vi "Get Error Type.vi"(1 "Newly Reported Error":T4, 2 "Last (latest) Handled Error":T2) -> (0 "Error Type":T1)   [LabVIEW 2023, in "Error Manager.lvlib"]
doc: "Blank VI with error handling."
uses:
  Error Manager.lvlib
  Reported Error (cluster).ctl
  Public API VIs/Pop-up New Error Dialogue Instruction (enum).ctl
  Handled Error (cluster).ctl
  Read-Unread Status (enum).ctl
  Error Log/Error Type (enum).ctl
  Error Log/Error Log.lvclass
panel:
  # "Input\nInputs to the VI"
  # "Development\nControls or indicators that are useful for development or testing, but which are not outputs of the VI."
  # "Output\nOutputs of the VI"
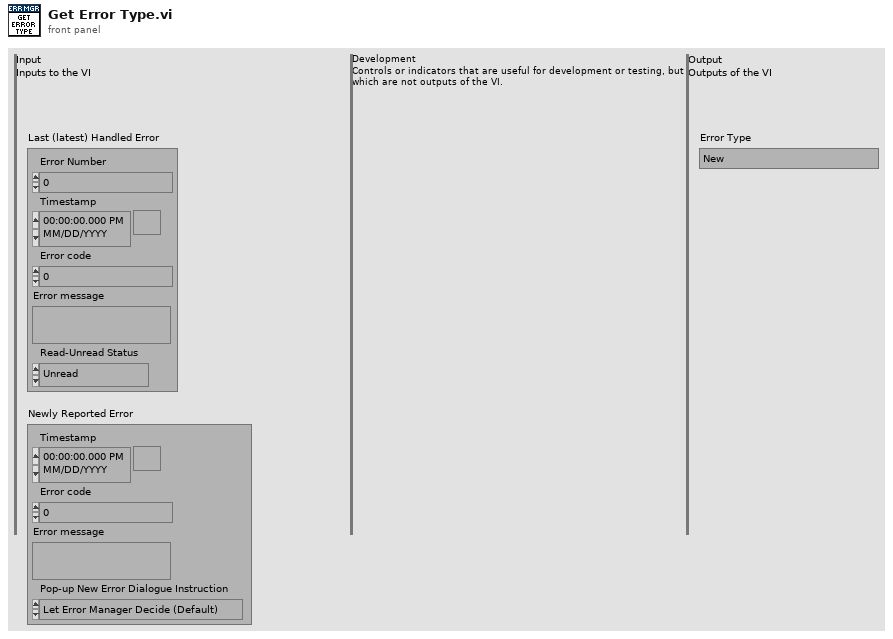
[diagram p1: front panel]
types:
  T1 = typedef "Error Manager.lvlib/Error Log.lvclass/Error Type (enum).ctl" = enum16{"New", "Identical to last logged error"}
  T2 = typedef "Error Manager.lvlib/Handled Error (cluster).ctl" = cluster{"Error Number":i32, "Timestamp":timestamp, "Error code":i32, "Error message":string, "Read-Unread Status":T3}
  T3 = typedef "Error Manager.lvlib/Read-Unread Status (enum).ctl" = enum16{"Unread", "Read"}
  T4 = typedef "Error Manager.lvlib/Reported Error (cluster).ctl" = cluster{"Timestamp":timestamp, "Error code":i32, "Error message":string, "Pop-up New Error Dialogue Instruction":T5}
  T5 = typedef "Error Manager.lvlib/Pop-up New Error Dialogue Instruction (enum).ctl" = enum16{"Let Error Manager Decide (Default)", "Don't pop-up", "Pop-up"}
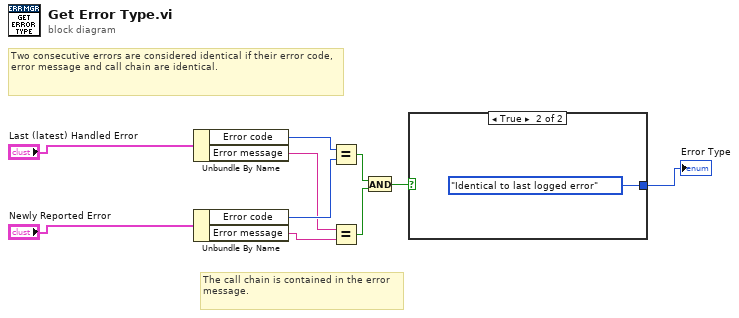
[diagram p0: block diagram]
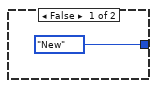
[diagram p2: hidden frame]
diagram:
  # "Two consecutive errors are considered identical if their error code, error message and call chain are identical."
  # "The call chain is contained in the error message."
  n1 = Unbundle By Name("Last (latest) Handled Error") -> ("Error code"=w8:i32, "Error message"=w6:string)
  n2 = Unbundle By Name("Newly Reported Error") -> ("Error code"=w7:i32, "Error message"=w5:string)
  n3 = Equal?(x=w8, y=w7) -> (x = y?=w4:bool)
  n4 = Equal?(x=w6, y=w5) -> (x = y?=w3:bool)
  n5 = And(x=w4, y=w3) -> (x .and. y?=w2:bool)
  n6 = case shown="True" w2 {
    tunnel: [Error_Type_(enum)."New" ("Error Type") Error_Type_(enum)."Identical to last logged error" ("Error Type")] -> w1
    frame False {
    }
    frame True {
    }
  }
  "Error Type" <- w1
